vi "Exemple_Metrics_Homogeneity_Completeness_V_Measure.vi"() -> ()   [LabVIEW 2020]
uses:
  Objet/3 - Model selection and evaluation/3.3 - Metrics and scoring/homogeneity_c_v_m/Homogeneity_C_V_M.vi
panel:
  out "Score":string
  out "error out":errorcluster caption="sortie d'erreur"
  in  "error in (no error)":errorcluster caption="entrée d'erreur (pas d'erreur)"
  in  "homogeneity_completeness_v_measure":cluster{"beta":dbl, "Returns":string}={"beta"=1.0, "Returns"="homogeneity"}
  in  "labels_pred":string[][](array[string])=[["1"], ["1"], ["0"], ["0"]]
  in  "labels_true":string[][](array[string])=[["0"], ["0"], ["1"], ["1"]]
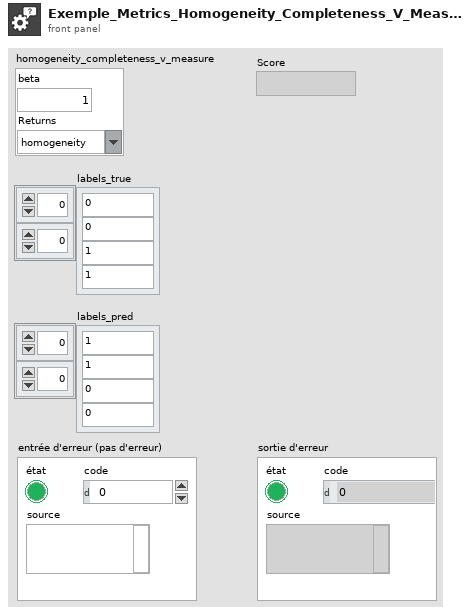
[diagram p1: front panel]
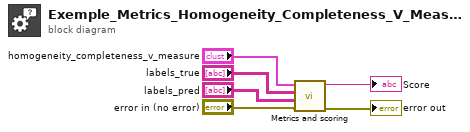
[diagram p0: block diagram]
diagram:
  n1 = call-poly "Metrics and scoring.vi"("error in (no error)"="error in (no error)", "labels_pred"="labels_pred", "labels_true"="labels_true", "homogeneity_completeness_v_measure"="homogeneity_completeness_v_measure") -> ("error out"=→"error out":errorcluster, "Score"=→"Score":string)  [unwired: 6 in]
